vi "Set OPC Ref.vi"(8 "error in (no error)":errorcluster, 10 "OPC UA server refnum":T1, 11 "Station in":refnum<class "Station.lvclass">) -> (0 "error out":errorcluster, 3 "Station out":refnum<class "Station.lvclass">)   [LabVIEW 2021]
uses:
  Station.lvclass
  C:/Program Files/National Instruments/LabVIEW 2021/vi.lib/ActorFramework/Actor/Actor.lvclass
  C:/GitHub/SM EOL OPC Server AF/Station/Station Actor/Station.lvclass
  <vilib>/OPCUA/controls/OPC UA Server Refnum.ctl
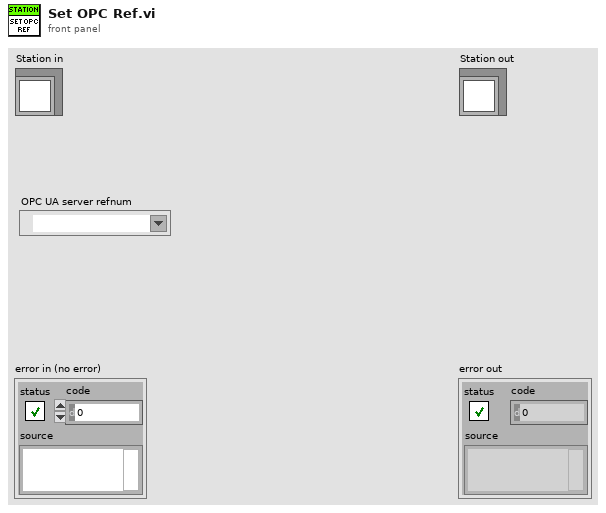
[diagram p1: front panel]
types:
  T1 = typedef "OPC UA Server Refnum.ctl" = refnum<k21>
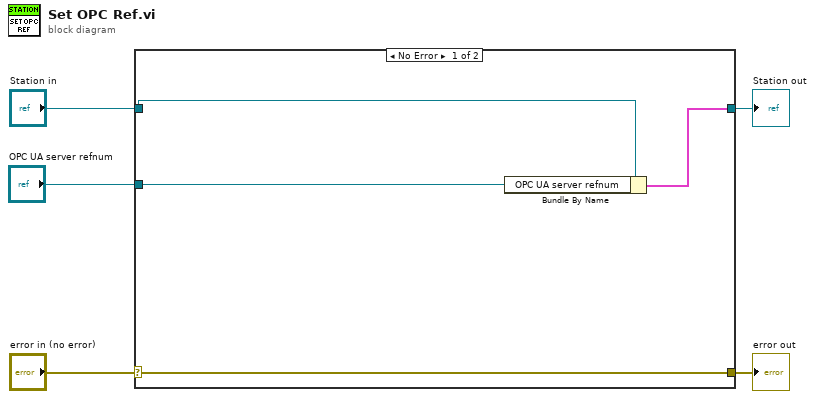
[diagram p0: block diagram]
diagram:
  n1 = case shown="No Error" "error in (no error)" {
    selector: "error in (no error)" -> [w9 w11]
    tunnel: [w9 w11] -> w4
    tunnel: [w7 w10] -> w2
    tunnel: "Station in" -> [w8 w10]
    tunnel: "OPC UA server refnum" -> [w6 _]
    frame No Error {
      n2 = Bundle By Name(cluster=w8, "OPC UA server refnum"=w6) -> (w7:cluster{})
    }
    frame Error {
    }
  }
  "error out" <- w4
  "Station out" <- w2
